vi "ChassisSpeeds_FromFieldRelativeChassisSpeeds.vi"(9 "RobotAngle":T2={"VALUE"=0.0, "COS"=1.0, "SIN"=0.0} {"SIN" format="%13.4f"; "COS" format="%13.4f"; "VALUE" format="%13.4f"}, 11 "FieldRelChassisSPeeds":T1 {"vOmega" format="%10.3f"; "vY" format="%10.3f"; "vX" format="%10.3f"}) -> (3 "CHASSIS":T1 {"vOmega" format="%10.3f"; "vY" format="%10.3f"; "vX" format="%10.3f"})   [LabVIEW 2019, in "Trajectory_Library.lvlib"]
doc: "Converts a user provided field-relative ChassisSpeeds object into a robot-relative ChassisSpeeds object.\n\n\n\nParameters: \n - fieldRelativeSpeeds -- The ChassisSpeeds object representing the speeds in the field frame\n of reference. Positive x is away from your alliance wall. Positive y is \n to your left when standing behind the alliance wall.\n - robotAngle -- The angle of the robot as measured by a gyroscope. The robot's angle is\n considered to be zero when it is facing directly away from your \n alliance station wall. Remember that this should be CCW positive.\n\nReturns:\n - ChassisSpeeds - Data structure representing the speeds in the robot's frame of reference."
uses:
  Trajectory_Library.lvlib
  TypeDef/CHASSIS_SPEEDS.ctl
  TypeDef/ROTATION2D.ctl
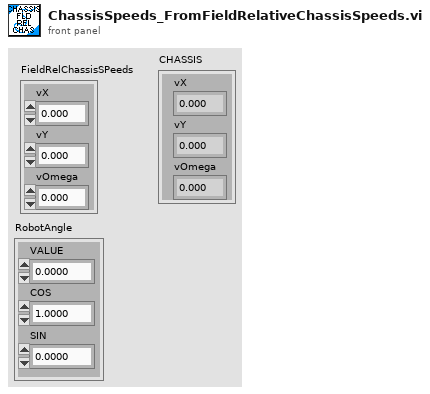
[diagram p1: front panel]
types:
  T1 = typedef "Trajectory_Library.lvlib/CHASSIS_SPEEDS.ctl" = cluster{"vX":dbl, "vY":dbl, "vOmega":dbl}
  T2 = typedef "Trajectory_Library.lvlib/ROTATION2D.ctl" = cluster{"VALUE":dbl, "COS":dbl, "SIN":dbl}
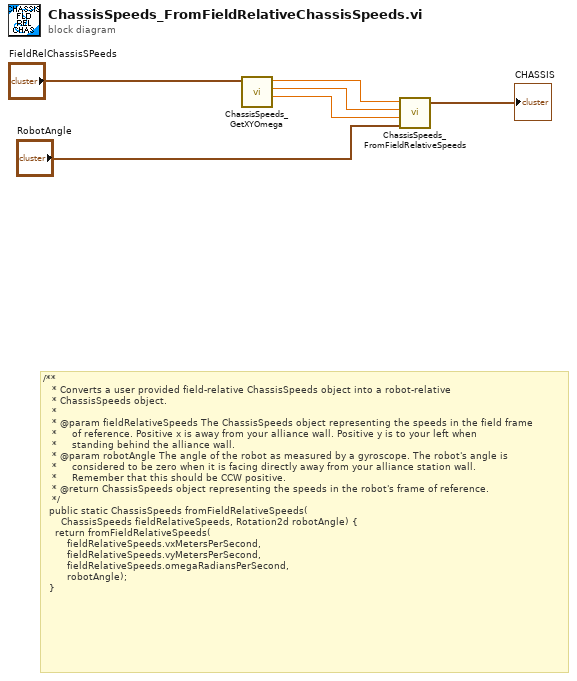
[diagram p0: block diagram]
diagram:
  # "/**\n   * Converts a user provided field-relative ChassisSpeeds object into a robot-relative\n   * ChassisSpeeds object.\n   *\n   * @param fieldRelativeSpeeds The ChassisSpeeds object representing the speeds in the field frame\n   *     of reference. Positive x is away from your alliance wall. Positive y is to your left when\n   *     standing behind the alliance wall.\n   * @param robotAngle The angle of the robot as measured by a gyroscope. The robot's angle is\n   *     considered to be zero when it is facing directly away from your alliance station wall.\n   *     Remember that this should be CCW positive.\n   * @return ChassisSpeeds object representing the speeds in the robot's frame of reference.\n   */\n  public static ChassisSpeeds fromFieldRelativeSpeeds(\n      ChassisSpeeds fieldRelativeSpeeds, Rotation2d robotAngle) {\n    return fromFieldRelativeSpeeds(\n        fieldRelativeSpeeds.vxMetersPerSecond,\n        fieldRelativeSpeeds.vyMetersPerSecond,\n        fieldRelativeSpeeds.omegaRadiansPerSecond,\n        robotAngle);\n  }"
  n1 = call "ChassisSpeeds_GetXYOmega.vi"("CHASSIS"="FieldRelChassisSPeeds") -> ("vAngular"=w2:dbl, "vY"=w3:dbl, "vX"=w4:dbl)  [unwired: 8 in]
  n2 = call "ChassisSpeeds_FromFieldRelativeSpeeds.vi"("RobotAngle"="RobotAngle", "Omega"=w2, "vY"=w3, "vX"=w4) -> ("CHASSIS"=→"CHASSIS":T1)  [unwired: 7 in]
